vi "Laser Feedback-v2.vi"() -> ()   [LabVIEW 2014]
doc: "This VI first scan 0.1-5 V AOM voltage range 3 times, and use these data to generate a calibration curve. The calibration curve is fitted as a 3 th order polynomial curve, and then passed to the second part. \nSecond, the feedback loop is turned on and PID controller is used to stabilize the intensity.\n\nThis VI includes the following subVI:\n1. (SubVI)AOMvolt-Power Calibration.vi\n2. AOM PID feedback-simplePID(SubVI).vi"
uses:
  <vilib>/DAQmx/create/channels.llb/DAQmx Create Channel (AO-Voltage-Basic).vi
  Main-Stage-PI/(Global) Current handle and LaserPower_YCC.vi
  <vilib>/Analysis/polynomials.llb/Scalar Polynomial Evaluation (DBL).vi
  <vilib>/addons/control/pid/pid.llb/PID (DBL).vi
  <vilib>/DAQmx/write.llb/DAQmx Write (Analog DBL 1Chan 1Samp).vi
  <vilib>/Analysis/NI_AALPro.lvlib
  <vilib>/addons/control/pid/NI_PID_pid.lvlib
panel:
  in  "File name add to the end":string="h300"
  out "time had recorded (s)":dbl
  in  "Record time (s)":dbl
  in  "Feedback?":bool=TRUE
  in  "Tab Control":enum32{"Calibration curve", "Power readout"}(tab)
  out "PW-AOM Graph":T1(graph)
  out "Waveform Chart":dbl(graph)
  out "Polynomial Coefficients":dbl[](array[numeric])
  out "AOM (V)":dbl format="%.2f"
  in  "Set Laser power":dbl
  out "Powermeter readout (mW)":dbl
  in  "Save Button":bool
  in  "PID gains 2":T2={"proportional gain (Kc)"=0.026000000000000002, "integral time (Ti, min)"=1.0000000000000011e-05, "derivative time (Td, min)"=0.0} {"derivative time (Td, min)" format="%#.6g"; "integral time (Ti, min)" format="%#.6g"; "proportional gain (Kc)" format="%#.6g"}
  in  "stop":bool
  in  "millisecond multiple":u32=1
  out "Start Calibrate":bool
  # "Kc=0.0151\nTi=2.1E-6\nTd=0.0093\n\nKc=0.0151\nTi=5E-6\nTd=0.0014"
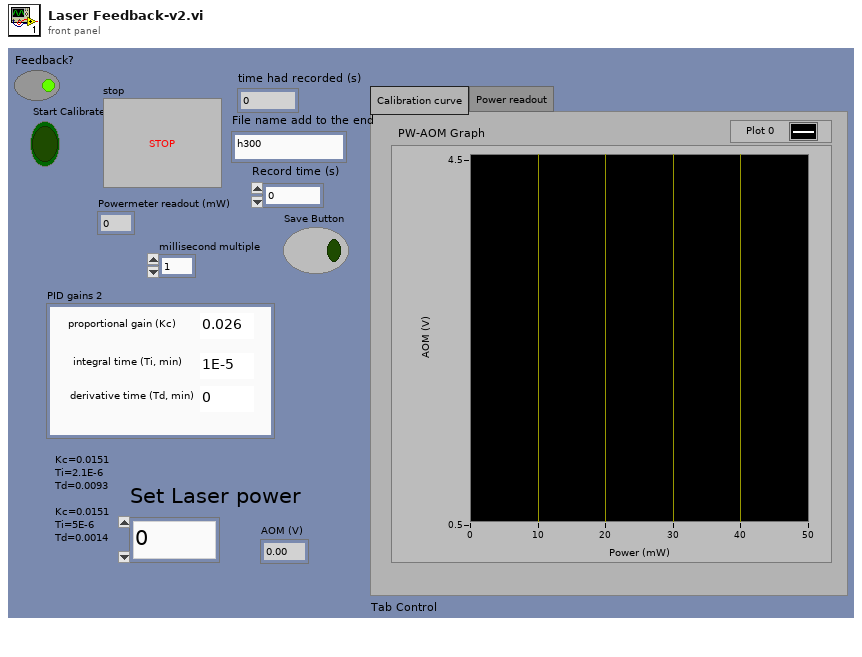
[diagram p1: front panel]
types:
  T1 = cluster{"Cal-PD (mV)":dbl[], "Cal-AOM (V)":dbl[]}[]
  T2 = cluster{"proportional gain (Kc)":dbl, "integral time (Ti, min)":dbl, "derivative time (Td, min)":dbl}
  T3 = cluster{"Cal-PD (mV)":dbl[], "Cal-AOM (V)":dbl[], "Best Polynomial Fit":dbl[], "Polynomial Coefficients":dbl[]}
  T4 = cluster{"Cal-PD (mV)":dbl[], "Best Polynomial Fit":dbl[]}
  T5 = cluster{"Cal-PD (mV)":dbl[], "Cal-AOM (V)":dbl[]}
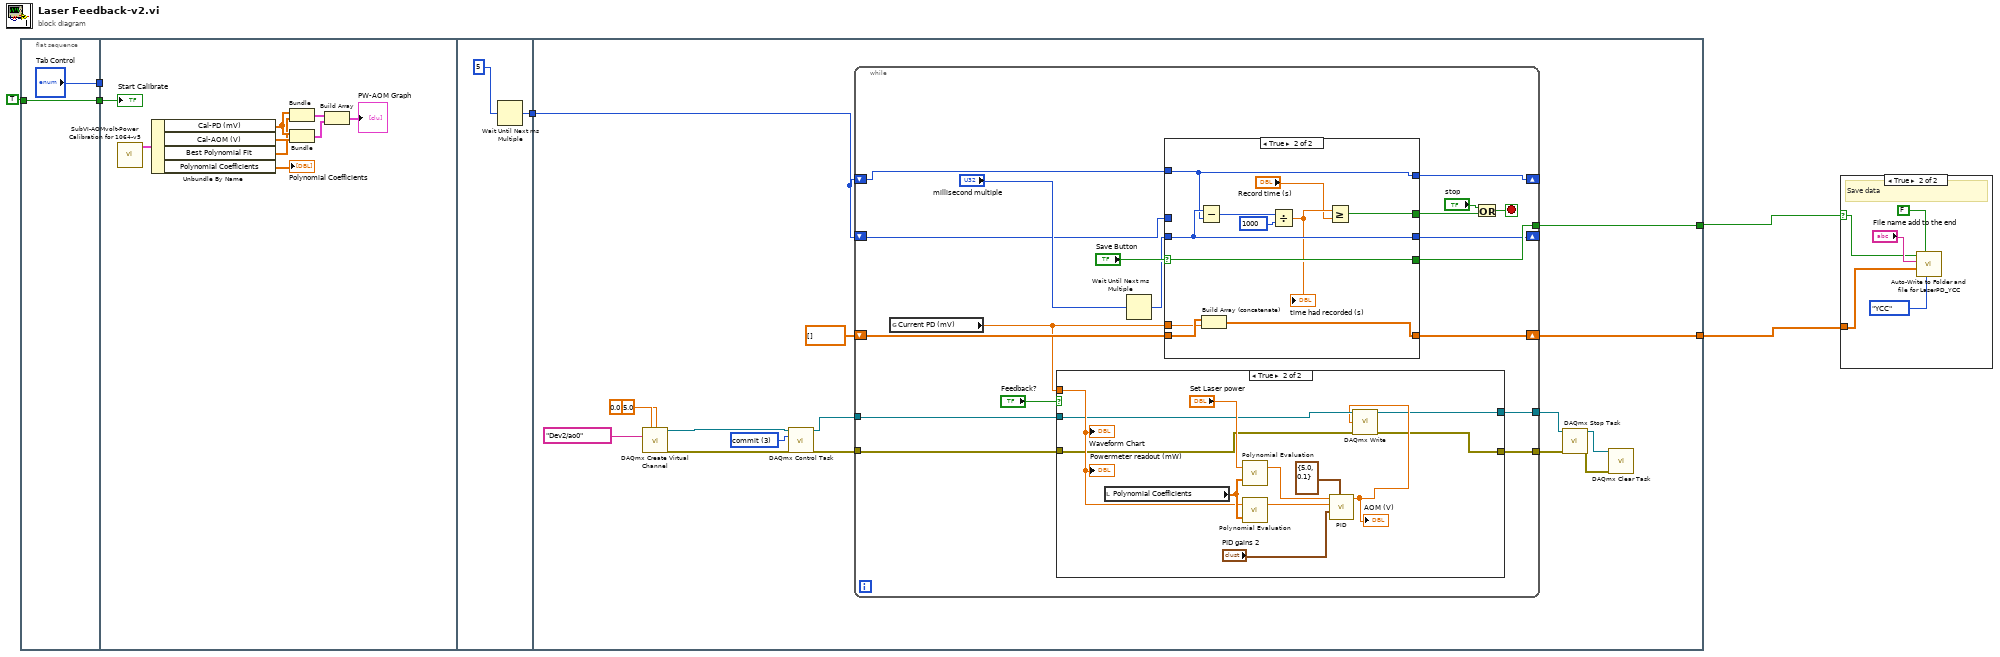
[diagram p0: block diagram]
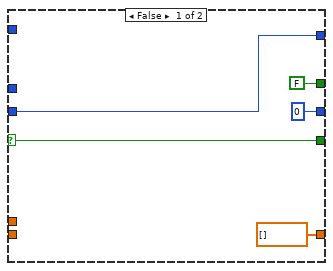
[diagram p4: hidden frame]
diagram:
  n1 = flat-sequence {
    tunnel: TRUE -> [w8]
    tunnel: [w8] -> w5
    tunnel: ["Tab Control"] -> w2
    tunnel: w5 -> [w17]
    tunnel: w2 -> [_]
    tunnel: [w18] -> w1
    tunnel: [w34] -> w4
    tunnel: [w33] -> w3
    tunnel: w1 -> [w32]
    frame #0 {
    }
    frame #1 {
      n2 = call "SubVI-AOMvolt-Power Calibration for 1064-v5.vi"() -> ("output cluster"=w16:T3)  [unwired: 7 in, 1 out]
      n3 = Unbundle By Name(w16) -> ("Cal-PD (mV)"=w13:dbl[], "Cal-AOM (V)"=w14:dbl[], "Best Polynomial Fit"=w12:dbl[], "Polynomial Coefficients"=→"Polynomial Coefficients":dbl[])
      n4 = Bundle("Cal-PD (mV)"=w13, "Best Polynomial Fit"=w12) -> (w11:T4)  [unwired: 1 in]
      n5 = Bundle("Cal-PD (mV)"=w13, "Cal-AOM (V)"=w14) -> (w10:T5)  [unwired: 1 in]
      n6 = Build Array(w11, w10) -> (→"PW-AOM Graph":T1)
      "Start Calibrate" <- w17
    }
    frame #2 {
      n7 = Wait Until Next ms Multiple(millisecond multiple=u32 5 ("milliseconds to wait")) -> (millisecond timer value=w18:u32)
    }
    frame #3 {
      w28 = 3 items=["verify"=2, "reserve"=4, "commit"=3, "unreserve"=5, "abort"=6] ("action")
      n8 = call-poly <vilib>:"DAQmx Create Virtual Channel.vi"("maximum value"=5.0, "minimum value"=0.0, "physical channels"=tag "Dev2/ao0") -> ("task out"=w29:refnum<k21>, "error out"=w30:errorcluster)  [unwired: 11 in]
      n9 = call <vilib>:"DAQmx Control Task.vi"("task/channels in"=w29, "action"=w28, "error in"=w30) -> ("task out"=w25:refnum<k21>, "error out"=w24:errorcluster)  [unwired: 11 in]
      n10 = while {
        tunnel: [w54] -> w34
        shift-right: [w53] -> w33
        shift-left: dbl[] [] -> [w52]
        shift-right: [w46] -> _
        shift-left: w32 -> [w45]
        shift-right: [w40] -> _
        shift-left: w32 -> [w41]
        tunnel: w25 -> [w39]
        tunnel: w24 -> [w38]
        tunnel: [w37] -> w23
        tunnel: [w36] -> w22
        stop <- w42 stop-if-true
        n11 = global read "(Global) Current handle and LaserPower_YCC.vi" "Current PD (mV)"() -> (w50:dbl)
        n12 = case shown="True" "Feedback?" {
          tunnel: w50 -> [_ w62]
          tunnel: w39 -> [w56 w61]
          tunnel: w38 -> [w55 w60]
          tunnel: [w56 w58] -> w37
          tunnel: [w55 w57] -> w36
          frame False {
          }
          frame True {
            n13 = local read "Polynomial Coefficients"() -> (w63:dbl[])
            n14 = call-poly <vilib>:"Polynomial Evaluation.vi"("P(x)"=w63, "a"="Set Laser power") -> ("P(a)"=w68:dbl)  [unwired: 1 out]
            n15 = call-poly <vilib>:"Polynomial Evaluation.vi"("P(x)"=w63, "a"=w62) -> ("P(a)"=w67:dbl)  [unwired: 1 out]
            n16 = call-poly <vilib>:"PID.vi"("output range"=cluster{"output high":dbl, "output low":dbl} {"output high"=5.0, "output low"=0.1}, "PID gains"="PID gains 2", "process variable"=w67, "setpoint"=w68) -> ("output"=w59:dbl)  [unwired: 6 in, 1 out]
            "AOM (V)" <- w59
            n17 = call-poly <vilib>:"DAQmx Write.vi"("task/channels in"=w61, "data"=w59, "error in"=w60) -> ("task out"=w58:refnum<k21>, "error out"=w57:errorcluster)  [unwired: 10 in, 1 out]
            "Powermeter readout (mW)" <- w62
            "Waveform Chart" <- w62
          }
        }
        n18 = Wait Until Next ms Multiple(millisecond multiple="millisecond multiple") -> (millisecond timer value=w47:u32)
        n19 = case shown="True" "Save Button" {
          selector: "Save Button" -> [w73 w84]
          tunnel: [w73 w84] -> w54
          tunnel: w50 -> [_ w82]
          tunnel: [dbl[] [] w81] -> w53
          tunnel: w52 -> [_ w83]
          tunnel: [u32 0 ("millisecond timer value") w80] -> w46
          tunnel: w47 -> [w70 w80]
          tunnel: w45 -> [_ _]
          tunnel: [FALSE w77] -> w44
          tunnel: w41 -> [_ w74]
          tunnel: [w70 w74] -> w40
          frame False {
          }
          frame True {
            n20 = Subtract(x=w80, y=w74) -> (x-y=w79:u32)
            n21 = Build Array (concatenate)(w83, w82) -> (w81:dbl[])
            n22 = Divide(x=w79, y=u32 1000) -> (x/y=w76:dbl)
            "time had recorded (s)" <- w76
            n23 = Greater Or Equal?(x=w76, y="Record time (s)") -> (x >= y?=w77:bool)
          }
        }
        n24 = Or(x="stop", y=w44) -> (x .or. y?=w42:bool)
      }
      n25 = call <vilib>:"DAQmx Stop Task.vi"("task/channels in"=w23, "error in"=w22) -> ("task out"=w21:refnum<k21>, "error out"=w20:errorcluster)  [unwired: 12 in]
      n26 = call <vilib>:"DAQmx Clear Task.vi"("task in"=w21, "error in"=w20) -> ()  [unwired: 13 in, 1 out]
    }
  }
  n27 = case shown="True" w4 {
    selector: w4 -> [_ w86]
    tunnel: w3 -> [_ w89]
    frame False {
    }
    frame True {
      # "Save data"
      n28 = call "Auto-Write to Folder and file for LaserPD_YCC.vi"("Who's Data"=enum16{"YCC", "PYW", "LCH", "YYH"}."YCC", "T=2D\nF=1D"=FALSE ("T=2D\nF=1D"), "1D data to be saved"=w89, "File name add to the end \n(height)"="File name add to the end", "Save?"=w86) -> ()  [unwired: 3 in, 2 out]
    }
  }
